vi "Read from file.vi"(11 "File Path":path) -> (3 "Data":T1)   [LabVIEW 2021]
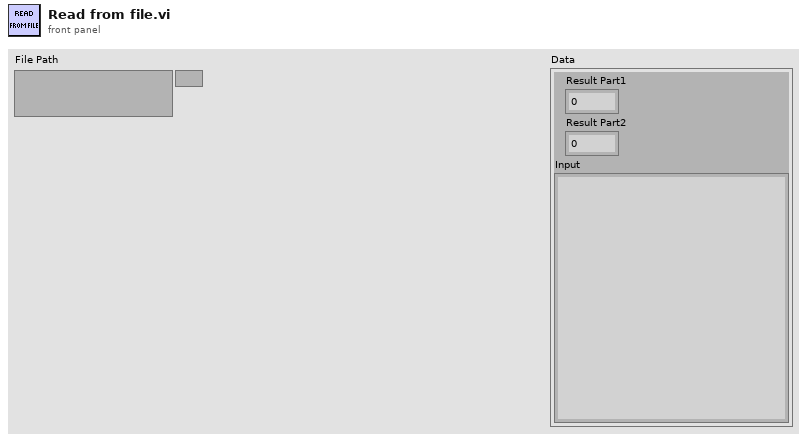
[diagram p1: front panel]
types:
  T1 = cluster{"Result Part1":dbl, "Result Part2":dbl, "Input":string}
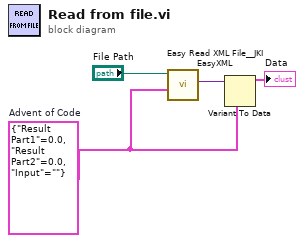
[diagram p0: block diagram]
diagram:
  w2 = T1 {"Result Part1"=0.0, "Result Part2"=0.0, "Input"=""}  # Advent of Code
  n1 = call <vilib>:"Easy Read XML File__JKI EasyXML.vi"("LabVIEW Data (Type)"=w2, "XML File Path"="File Path") -> ("LabVIEW Data"=w3:variant)  [unwired: 7 in, 2 out]
  n2 = Variant To Data(type=w2, Variant=w3) -> (data=→"Data":T1)  [unwired: 1 in, 1 out]
